vi "Set MES Enabled.vi"(8 "error in (no error)":errorcluster, 10 "MES Enabled":bool, 11 "App Settings in":refnum<class "App Settings.lvclass">) -> (0 "error out":errorcluster, 3 "App Settings out":refnum<class "App Settings.lvclass">)   [LabVIEW 2017]
uses:
  App Settings.lvclass
  C:/Test System Services/Acrobat Framework/ACRObat Test Framework/Main Framework/Release/Test Framework/Classes/Base Objects/Base Class/Base Class/Class Settings/Class Settings.lvclass
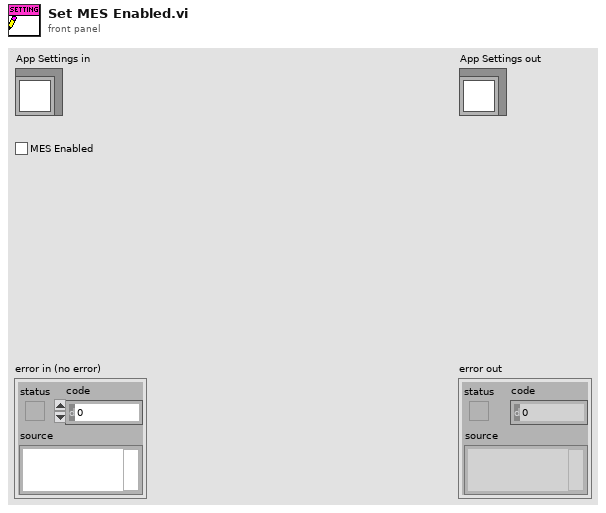
[diagram p1: front panel]
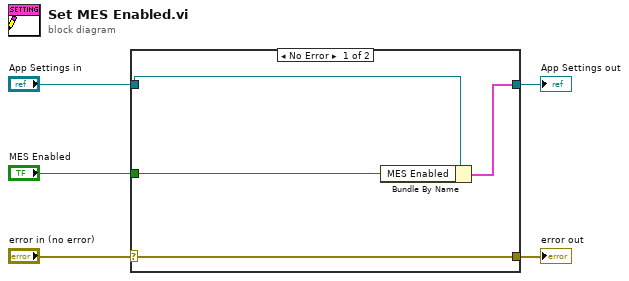
[diagram p0: block diagram]
diagram:
  n1 = case shown="No Error" "error in (no error)" {
    selector: "error in (no error)" -> [w9 w10]
    tunnel: [w9 w10] -> w4
    tunnel: [w7 w11] -> w2
    tunnel: "App Settings in" -> [w8 w11]
    tunnel: "MES Enabled" -> [w6 _]
    frame No Error {
      n2 = Bundle By Name(cluster=w8, "MES Enabled"=w6) -> (w7:cluster{})
    }
    frame Error {
    }
  }
  "error out" <- w4
  "App Settings out" <- w2
